vi "output.vi"(8 "error in":errorcluster, 10 "data table in":T1, 11 "UI Reference runtime in":refnum<class "UI Reference runtime.lvclass">) -> (0 "error out":errorcluster, 2 "data table out":T1, 3 "UI Reference runtime out":refnum<class "UI Reference runtime.lvclass">)   [LabVIEW 2013, in "UI Reference runtime.lvclass"]
doc: "Provides an interface for writing data to a module at runtime. While this interface performs no operations, a child should provide an override which may write to any open sessions, references, or interfaces."
uses:
  UI Reference runtime.lvclass
  <vilib>/NI/Tag Bus/table/data table.ctl
  UI Reference runtime.lvclass/UI Reference runtime.ctl
  <vilib>/NI/Tag Bus/table/data polymorphs/read many/read Doubles.vi
  <vilib>/NI/Tag Bus/table/data polymorphs/read many/read Singles.vi
  <vilib>/NI/Tag Bus/table/data polymorphs/read many/read I64s.vi
  <vilib>/NI/Tag Bus/table/data polymorphs/read many/read I32s.vi
  <vilib>/NI/Tag Bus/table/data polymorphs/read many/read I16s.vi
  <vilib>/NI/Tag Bus/table/data polymorphs/read many/read I8s.vi
  <vilib>/NI/Tag Bus/table/data polymorphs/read many/read U64s.vi
  <vilib>/NI/Tag Bus/table/data polymorphs/read many/read U32s.vi
  <vilib>/NI/Tag Bus/table/data polymorphs/read many/read U16s.vi
  <vilib>/NI/Tag Bus/table/data polymorphs/read many/read U8s.vi
  <vilib>/NI/Tag Bus/table/data polymorphs/read many/read Booleans.vi
  <vilib>/NI/Tag Bus/table/data polymorphs/read many/read Strings.vi
  <vilib>/NI/Tag Bus/table/data polymorphs/read one/read Array of Double.vi
  <vilib>/NI/Tag Bus/table/data polymorphs/read one/read Array of Single.vi
  <vilib>/NI/Tag Bus/table/data polymorphs/read one/read Array of I64.vi
  <vilib>/NI/Tag Bus/table/data polymorphs/read one/read Array of I32.vi
  <vilib>/NI/Tag Bus/table/data polymorphs/read one/read Array of I16.vi
  <vilib>/NI/Tag Bus/table/data polymorphs/read one/read Array of I8.vi
  <vilib>/NI/Tag Bus/table/data polymorphs/read one/read Array of U64.vi
  <vilib>/NI/Tag Bus/table/data polymorphs/read one/read Array of U32.vi
  <vilib>/NI/Tag Bus/table/data polymorphs/read one/read Array of U16.vi
  <vilib>/NI/Tag Bus/table/data polymorphs/read one/read Array of U8.vi
  <vilib>/NI/Tag Bus/table/data polymorphs/read one/read Array of Boolean.vi
  <vilib>/NI/Tag Bus/table/data polymorphs/read one/read Array of String.vi
  <vilib>/NI/Tag Bus/table/data table.lvlib
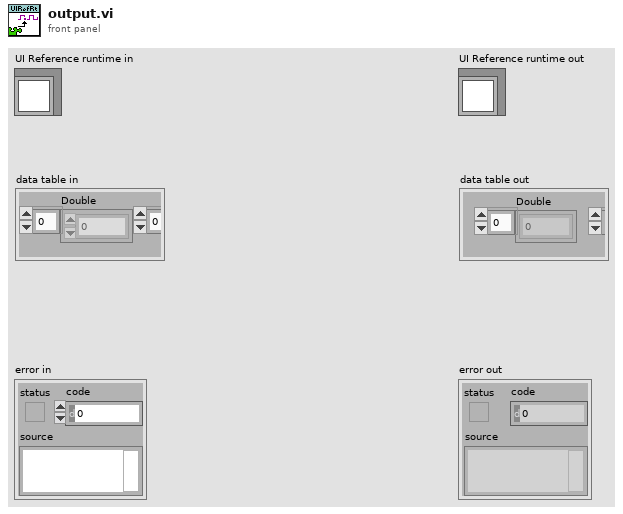
[diagram p1: front panel]
types:
  T1 = typedef "tag bus.lvlib/data table.lvlib/data table.ctl" = cluster{"Double":dbl[], "Single":sgl[], "I64":i64[], "I32":i32[], "I16":i16[], "I8":i8[], "U64":u64[], "U32":u32[], "U16":u16[], "U8":u8[], "Boolean":bool[], "String":string[], "Array of Double":cluster{"DBL Array":dbl[]}[], "Array of Single":cluster{"SGL Array":sgl[]}[], "Array of I64":cluster{"I64 Array":i64[]}[], "Array of I32":cluster{"I32 Array":i32[]}[], "Array of I16":cluster{"I16 Array":i16[]}[], "Array of I8":cluster{"I8 Array":i8[]}[], "Array of U64":cluster{"U64 Array":u64[]}[], "Array of U32":cluster{"U32 Array":u32[]}[], "Array of U16":cluster{"U16 Array":u16[]}[], "Array of U8":cluster{"U8 Array":u8[]}[], "Array of Boolean":cluster{"Boolean Array":bool[]}[], "Array of String":cluster{"String Array":string[]}[]}
  T2 = typedef "UI Reference runtime.lvclass/control index set.ctl" = cluster{"data type":T3, "control indexes":i32[], "data indexes":i32[]}
  T3 = typedef "tag bus.lvlib/tag descriptor.lvclass/Data Type.ctl" = enum16{"Double", "Single", "I64", "I32", "I16", "I8", "U64", "U32", "U16", "U8", "Boolean", "String", "Array of Double", "Array of Single", "Array of I64", "Array of I32", "Array of I16", "Array of I8", "Array of U64", "Array of U32", "Array of U16", "Array of U8", "Array of Boolean", "Array of String"}
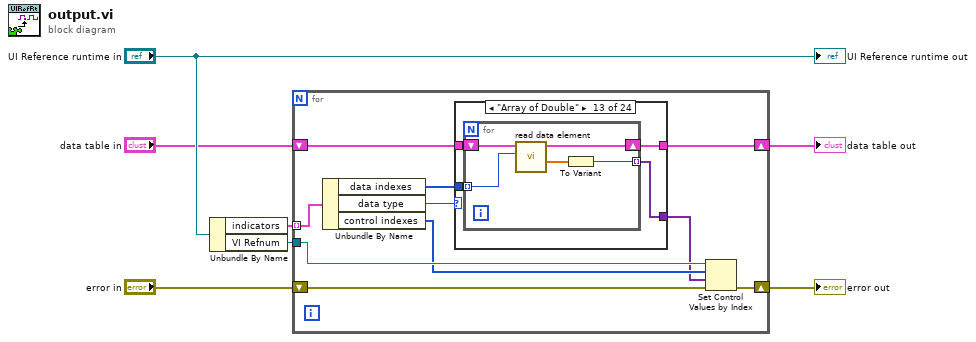
[diagram p0: block diagram]
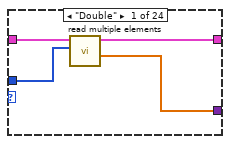
[diagram p2: hidden frame]
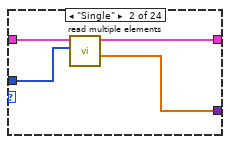
[diagram p3: hidden frame]
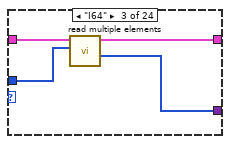
[diagram p4: hidden frame]
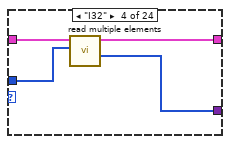
[diagram p5: hidden frame]
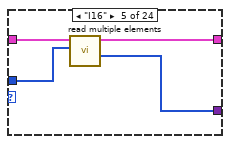
[diagram p6: hidden frame]
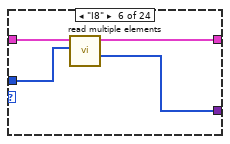
[diagram p7: hidden frame]
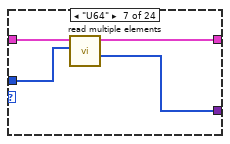
[diagram p8: hidden frame]
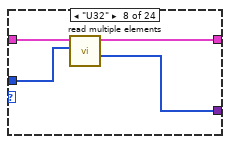
[diagram p9: hidden frame]
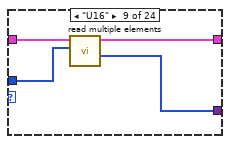
[diagram p10: hidden frame]
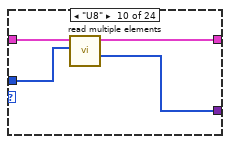
[diagram p11: hidden frame]
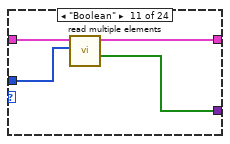
[diagram p12: hidden frame]
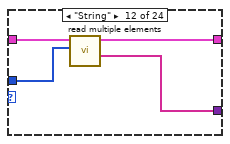
[diagram p13: hidden frame]
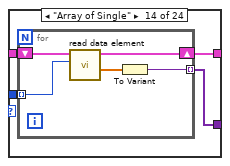
[diagram p14: hidden frame]
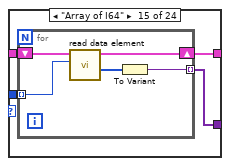
[diagram p15: hidden frame]
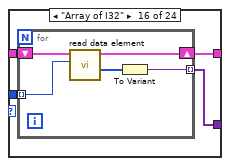
[diagram p16: hidden frame]
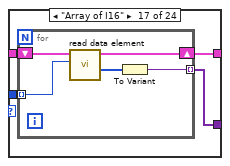
[diagram p17: hidden frame]
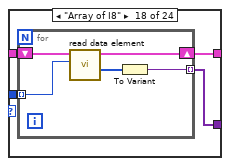
[diagram p18: hidden frame]
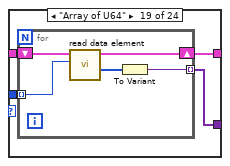
[diagram p19: hidden frame]
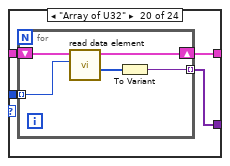
[diagram p20: hidden frame]
diagram:
  n1 = Unbundle By Name("UI Reference runtime in") -> ("indicators"=w7:T2[], "VI Refnum"=w6:refnum<vi>)
  n2 = for {
    shift-right: [w11] -> w2
    shift-left: "data table in" -> [w10]
    shift-right: [w16] -> w4
    shift-left: "error in" -> [w15]
    tunnel: w7 -> [w17] mode=indexing
    tunnel: w6 -> [w14]
    n3 = Unbundle By Name(w17) -> ("data indexes"=w9:i32[], "data type"=w12:T3, "control indexes"=w13:i32[])
    n4 = case shown="\"Array of Double\"" w12 {
      tunnel: [w20 w24 w28 w32 w36 w40 w44 w48 w52 w56 w60 w64 w68 w77 w86 w95 w104 w113 w122 w131 w140 w149 w158 w167] -> w11
      tunnel: w10 -> [w21 w25 w29 w33 w37 w41 w45 w49 w53 w57 w61 w65 w69 w78 w87 w96 w105 w114 w123 w132 w141 w150 w159 w168]
      tunnel: w9 -> [w19 w23 w27 w31 w35 w39 w43 w47 w51 w55 w59 w63 w67 w76 w85 w94 w103 w112 w121 w130 w139 w148 w157 w166]
      tunnel: [w18 w22 w26 w30 w34 w38 w42 w46 w50 w54 w58 w62 w66 w75 w84 w93 w102 w111 w120 w129 w138 w147 w156 w165] -> w8
      frame "Double" {
        n5 = call-poly <vilib>:"read multiple elements.vi"("indices"=w19, "data table in"=w21) -> ("values"=w18:dbl[], "data table out"=w20:T1)  [unwired: 8 in]
      }
      frame "Single" {
        n6 = call-poly <vilib>:"read multiple elements.vi"("indices"=w23, "data table in"=w25) -> ("values"=w22:sgl[], "data table out"=w24:T1)  [unwired: 8 in]
      }
      frame "I64" {
        n7 = call-poly <vilib>:"read multiple elements.vi"("indices"=w27, "data table in"=w29) -> ("values"=w26:i64[], "data table out"=w28:T1)  [unwired: 8 in]
      }
      frame "I32" {
        n8 = call-poly <vilib>:"read multiple elements.vi"("indices"=w31, "data table in"=w33) -> ("values"=w30:i32[], "data table out"=w32:T1)  [unwired: 8 in]
      }
      frame "I16" {
        n9 = call-poly <vilib>:"read multiple elements.vi"("indices"=w35, "data table in"=w37) -> ("values"=w34:i16[], "data table out"=w36:T1)  [unwired: 8 in]
      }
      frame "I8" {
        n10 = call-poly <vilib>:"read multiple elements.vi"("indices"=w39, "data table in"=w41) -> ("values"=w38:i8[], "data table out"=w40:T1)  [unwired: 8 in]
      }
      frame "U64" {
        n11 = call-poly <vilib>:"read multiple elements.vi"("indices"=w43, "data table in"=w45) -> ("values"=w42:u64[], "data table out"=w44:T1)  [unwired: 8 in]
      }
      frame "U32" {
        n12 = call-poly <vilib>:"read multiple elements.vi"("indices"=w47, "data table in"=w49) -> ("values"=w46:u32[], "data table out"=w48:T1)  [unwired: 8 in]
      }
      frame "U16" {
        n13 = call-poly <vilib>:"read multiple elements.vi"("indices"=w51, "data table in"=w53) -> ("values"=w50:u16[], "data table out"=w52:T1)  [unwired: 8 in]
      }
      frame "U8" {
        n14 = call-poly <vilib>:"read multiple elements.vi"("indices"=w55, "data table in"=w57) -> ("values"=w54:u8[], "data table out"=w56:T1)  [unwired: 8 in]
      }
      frame "Boolean" {
        n15 = call-poly <vilib>:"read multiple elements.vi"("indices"=w59, "data table in"=w61) -> ("values"=w58:bool[], "data table out"=w60:T1)  [unwired: 8 in]
      }
      frame "String" {
        n16 = call-poly <vilib>:"read multiple elements.vi"("indices"=w63, "data table in"=w65) -> ("values"=w62:string[], "data table out"=w64:T1)  [unwired: 8 in]
      }
      frame "Array of Double" {
        n17 = for {
          tunnel: w67 -> [w72] mode=indexing
          tunnel: [w70] -> w66 mode=indexing
          shift-right: [w73] -> w68
          shift-left: w69 -> [w74]
          n18 = call-poly <vilib>:"read data element.vi"("index"=w72, "data table in"=w74) -> ("value"=w71:dbl[], "data table out"=w73:T1)  [unwired: 8 in]
          n19 = To Variant(anything=w71) -> (Variant=w70:variant)
        }
      }
      frame "Array of Single" {
        n20 = for {
          tunnel: w76 -> [w81] mode=indexing
          tunnel: [w79] -> w75 mode=indexing
          shift-right: [w82] -> w77
          shift-left: w78 -> [w83]
          n21 = call-poly <vilib>:"read data element.vi"("index"=w81, "data table in"=w83) -> ("value"=w80:sgl[], "data table out"=w82:T1)  [unwired: 8 in]
          n22 = To Variant(anything=w80) -> (Variant=w79:variant)
        }
      }
      frame "Array of I64" {
        n23 = for {
          tunnel: w85 -> [w90] mode=indexing
          tunnel: [w88] -> w84 mode=indexing
          shift-right: [w91] -> w86
          shift-left: w87 -> [w92]
          n24 = call-poly <vilib>:"read data element.vi"("index"=w90, "data table in"=w92) -> ("value"=w89:i64[], "data table out"=w91:T1)  [unwired: 8 in]
          n25 = To Variant(anything=w89) -> (Variant=w88:variant)
        }
      }
      frame "Array of I32" {
        n26 = for {
          tunnel: w94 -> [w99] mode=indexing
          tunnel: [w97] -> w93 mode=indexing
          shift-right: [w100] -> w95
          shift-left: w96 -> [w101]
          n27 = call-poly <vilib>:"read data element.vi"("index"=w99, "data table in"=w101) -> ("value"=w98:i32[], "data table out"=w100:T1)  [unwired: 8 in]
          n28 = To Variant(anything=w98) -> (Variant=w97:variant)
        }
      }
      frame "Array of I16" {
        n29 = for {
          tunnel: w103 -> [w108] mode=indexing
          tunnel: [w106] -> w102 mode=indexing
          shift-right: [w109] -> w104
          shift-left: w105 -> [w110]
          n30 = call-poly <vilib>:"read data element.vi"("index"=w108, "data table in"=w110) -> ("value"=w107:i16[], "data table out"=w109:T1)  [unwired: 8 in]
          n31 = To Variant(anything=w107) -> (Variant=w106:variant)
        }
      }
      frame "Array of I8" {
        n32 = for {
          tunnel: w112 -> [w117] mode=indexing
          tunnel: [w115] -> w111 mode=indexing
          shift-right: [w118] -> w113
          shift-left: w114 -> [w119]
          n33 = call-poly <vilib>:"read data element.vi"("index"=w117, "data table in"=w119) -> ("value"=w116:i8[], "data table out"=w118:T1)  [unwired: 8 in]
          n34 = To Variant(anything=w116) -> (Variant=w115:variant)
        }
      }
      frame "Array of U64" {
        n35 = for {
          tunnel: w121 -> [w126] mode=indexing
          tunnel: [w124] -> w120 mode=indexing
          shift-right: [w127] -> w122
          shift-left: w123 -> [w128]
          n36 = call-poly <vilib>:"read data element.vi"("index"=w126, "data table in"=w128) -> ("value"=w125:u64[], "data table out"=w127:T1)  [unwired: 8 in]
          n37 = To Variant(anything=w125) -> (Variant=w124:variant)
        }
      }
      frame "Array of U32" {
        n38 = for {
          tunnel: w130 -> [w135] mode=indexing
          tunnel: [w133] -> w129 mode=indexing
          shift-right: [w136] -> w131
          shift-left: w132 -> [w137]
          n39 = call-poly <vilib>:"read data element.vi"("index"=w135, "data table in"=w137) -> ("value"=w134:u32[], "data table out"=w136:T1)  [unwired: 8 in]
          n40 = To Variant(anything=w134) -> (Variant=w133:variant)
        }
      }
      frame "Array of U16" {
        n41 = for {
          tunnel: w139 -> [w144] mode=indexing
          tunnel: [w142] -> w138 mode=indexing
          shift-right: [w145] -> w140
          shift-left: w141 -> [w146]
          n42 = call-poly <vilib>:"read data element.vi"("index"=w144, "data table in"=w146) -> ("value"=w143:u16[], "data table out"=w145:T1)  [unwired: 8 in]
          n43 = To Variant(anything=w143) -> (Variant=w142:variant)
        }
      }
      frame "Array of U8" {
        n44 = for {
          tunnel: w148 -> [w153] mode=indexing
          tunnel: [w151] -> w147 mode=indexing
          shift-right: [w154] -> w149
          shift-left: w150 -> [w155]
          n45 = call-poly <vilib>:"read data element.vi"("index"=w153, "data table in"=w155) -> ("value"=w152:u8[], "data table out"=w154:T1)  [unwired: 8 in]
          n46 = To Variant(anything=w152) -> (Variant=w151:variant)
        }
      }
      frame "Array of Boolean" {
        n47 = for {
          tunnel: w157 -> [w162] mode=indexing
          tunnel: [w160] -> w156 mode=indexing
          shift-right: [w163] -> w158
          shift-left: w159 -> [w164]
          n48 = call-poly <vilib>:"read data element.vi"("index"=w162, "data table in"=w164) -> ("value"=w161:bool[], "data table out"=w163:T1)  [unwired: 8 in]
          n49 = To Variant(anything=w161) -> (Variant=w160:variant)
        }
      }
      frame "Array of String" {
        n50 = for {
          tunnel: w166 -> [w171] mode=indexing
          tunnel: [w169] -> w165 mode=indexing
          shift-right: [w172] -> w167
          shift-left: w168 -> [w173]
          n51 = call-poly <vilib>:"read data element.vi"("index"=w171, "data table in"=w173) -> ("value"=w170:string[], "data table out"=w172:T1)  [unwired: 8 in]
          n52 = To Variant(anything=w170) -> (Variant=w169:variant)
        }
      }
    }
    n53 = Set Control Values by Index(0:w14, 1:w13, 2:w8, 3:w15) -> (11:w16:errorcluster)
  }
  "error out" <- w4
  "data table out" <- w2
  "UI Reference runtime out" <- "UI Reference runtime in"
